vi "WSVCAP SHL Host TL I2C Read - Single Device.vi"(0 "Bytes to Read (1-4)":u8=4 min=1 max=4 step=1, 3 "FPGA":T1, 5 "Sub Address [U8]":u8=191 format="%.0x", 11 "error in":errorcluster, 12 "DUT":T2, 14 "Log (T)":bool=TRUE) -> (4 "Device Data":u8[](array[numeric]) format="%.0x", 15 "error out":errorcluster)   [LabVIEW 2017]
uses:
  Type Defs/WSVCAP SHL DUT Number Enum.ctl
  Type Defs/WSVCAP SHL FPGA Enum.ctl
panel:
  out "Socket Mask [U64]":u64 format="%012x"
  out "C1:1-24 Read Data [U8]":u8[][](array[numeric]) format="%.0x"
  out "Data Headers":u8[](array[numeric])=[1, 2, 3, 4, 5, 6, 7, 8, 9, 10, 11, 12, 12, 14, 15, 16, 17, 18, 19, 20, 21, 22, 23, 24, 25, 26, 27, 28, 29, 30, 31, 32, 33, 34, 35, 36]
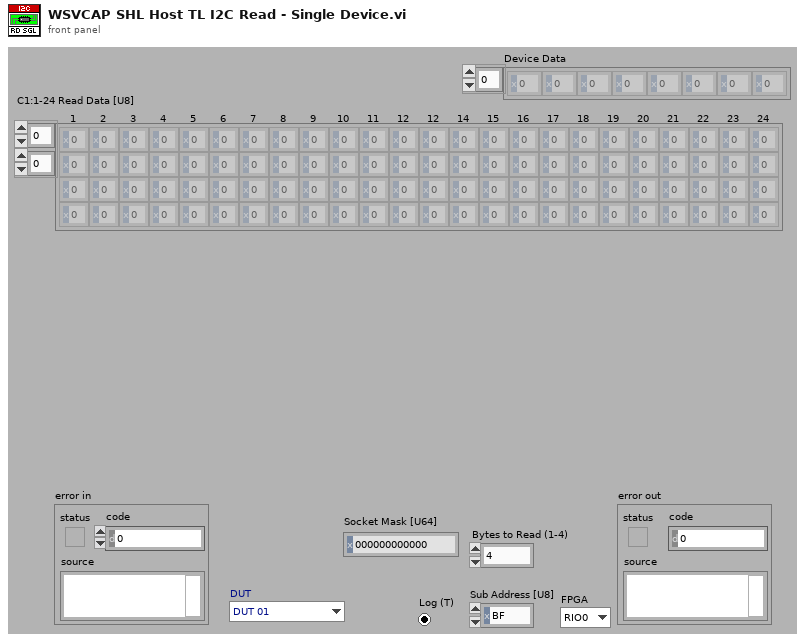
[diagram p1: front panel]
types:
  T1 = typedef "WSVCAP SHL FPGA Enum.ctl" = enum16{"RIO0", "RIO1"}
  T2 = typedef "WSVCAP SHL DUT Number Enum.ctl" = enum16{"DUT 01", "DUT 02", "DUT 03", "DUT 04", "DUT 05", "DUT 06", "DUT 07", "DUT 08", "DUT 09", "DUT 10", "DUT 11", "DUT 12", "DUT 13", "DUT 14", "DUT 15", "DUT 16", "DUT 17", "DUT 18", "DUT 19", "DUT 20", "DUT 21", "DUT 22", "DUT 23", "DUT 24", "DUT 25", "DUT 26", "DUT 27", "DUT 28", "DUT 29", "DUT 30", "DUT 31", "DUT 32", "DUT 33", "DUT 34", "DUT 35", "DUT 36", "DUT 37", "DUT 38", "DUT 39", "DUT 40", "DUT 41", "DUT 42", "DUT 43", "DUT 44", "DUT 45", "DUT 46", "DUT 47", "DUT 48", "DUT 49", "DUT 50", "DUT 51", "DUT 52", "DUT 53", "DUT 54", "DUT 55", "DUT 56", "DUT 57", "DUT 58", "DUT 59", "DUT 60", "DUT 61", "DUT 62", "DUT 63", "DUT 64"}
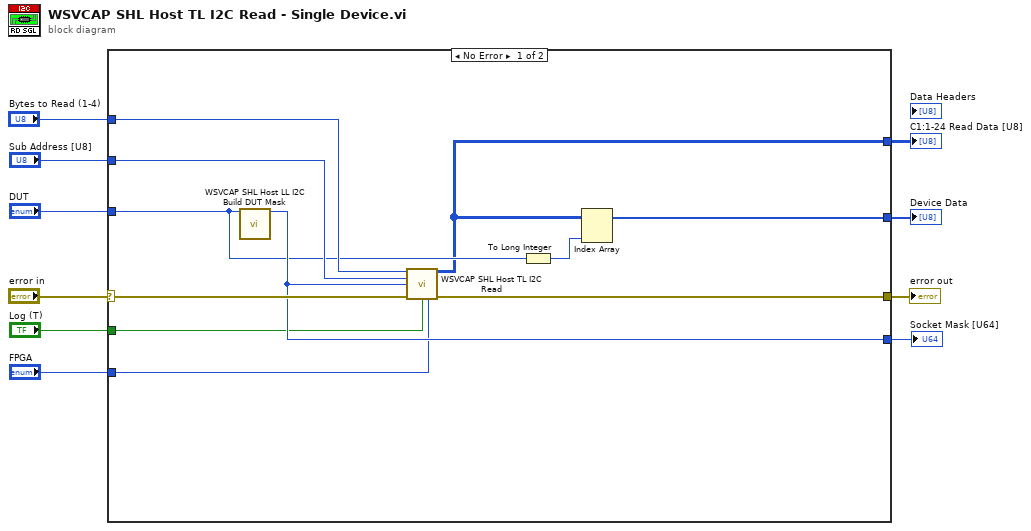
[diagram p0: block diagram]
diagram:
  n1 = case shown="No Error" "error in" {
    selector: "error in" -> [w20 w22]
    tunnel: [w21 w22] -> w10
    tunnel: "Bytes to Read (1-4)" -> [w19 _]
    tunnel: "Sub Address [U8]" -> [w18 _]
    tunnel: "DUT" -> [w14 _]
    tunnel: [w17 _] -> w5
    tunnel: [w12 _] -> w4
    tunnel: [w16 _] -> w3
    tunnel: "Log (T)" -> [w15 _]
    tunnel: "FPGA" -> [w13 _]
    frame No Error {
      n2 = call "WSVCAP SHL Host LL I2C Build DUT Mask.vi"("DUT"=w14) -> ("Socket Mask [U64]"=w17:u64)  [unwired: 13 in, 1 out]
      n3 = call "WSVCAP SHL Host TL I2C Read.vi"("Bytes to Read"=w19, "Sub Address [U8]"=w18, "Socket Mask [U64]"=w17, "error in"=w20, "Log (T)"=w15, "FPGA"=w13) -> ("C Read Data Out"=w12:u8[][], "error out"=w21:errorcluster)  [unwired: 8 in]
      n4 = To Long Integer(number=w14) -> (32bit integer=w11:i32)
      n5 = Index Array(array=w12, index (col)=w11) -> (element=w16:u8[])  [unwired: 1 in]
    }
    frame Error {
    }
  }
  "error out" <- w10
  "Socket Mask [U64]" <- w5
  "C1:1-24 Read Data [U8]" <- w4
  "Device Data" <- w3
